vi "1.1 比大小.vi"() -> ()   [LabVIEW 2022 SP3]
panel:
  in  "停止":bool
  out "布尔":bool
  in  "数值 2":dbl
  in  "数值":dbl
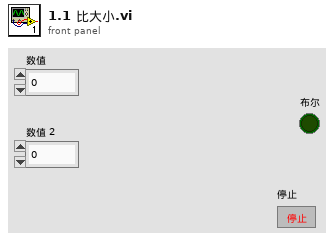
[diagram p1: front panel]
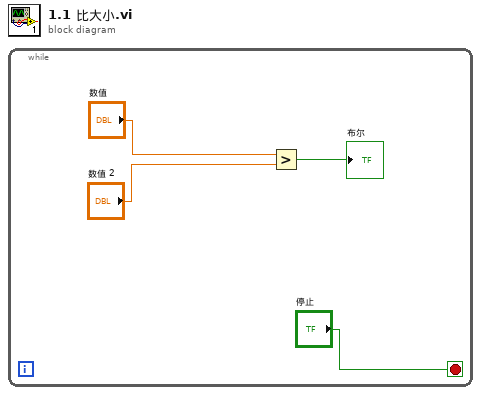
[diagram p0: block diagram]
diagram:
  n1 = while {
    stop <- "停止" stop-if-true
    n2 = Greater?(x="数值", y="数值 2") -> (0:→"布尔":bool)
  }
